vi "SystemController.UIClosed.vi"(8 "error in (no error)":errorcluster, 10 "UIClosed":T1, 11 "SystemController":refnum<class "SystemController.lvclass">) -> (0 "error out":errorcluster, 3 "SystemController out":refnum<class "SystemController.lvclass">)   [LabVIEW 2017, in "SystemController.lvclass"]
doc: "---------------------------------------------------------------\nJKI State Machine Objects™\nhttp://jki.net/state-machine-objects/\nCopyright (C) 2005-2015, JKI <info@jki.net>\nALL RIGHTS RESERVEDJKI State Machine Objects (SMO) 1.0.0.4\nJKI - JKI\nCopyright (c) 2015, JKI"
uses:
  SystemController.lvclass
  Typedefs/PublicEvents--SystemController.UIClosed.ctl
  SystemController.lvclass/SystemController.ctl
panel:
  # "For instructions on how to use the JKI State Machine Objects, examples and video tutorials, visit:\nhttp://jki.net/state-machine-objects/\n\nJKI State Machine Objects™\nhttp://jki.net/state-machine-objects/\nCopyright (C) 2005-2015, JKI <info@jki.net>\nALL RIGHTS RESERVED"
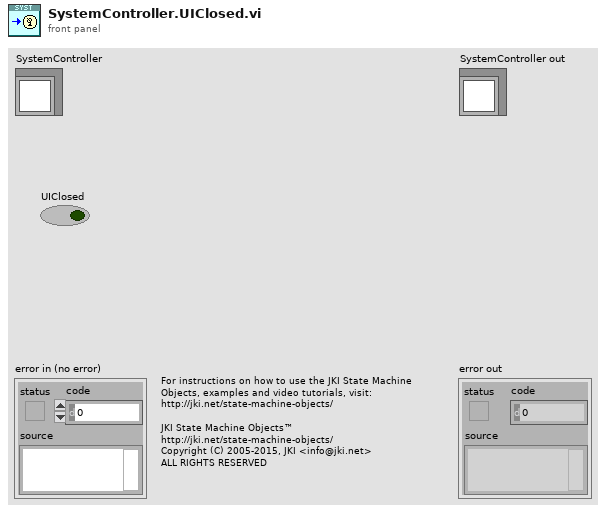
[diagram p1: front panel]
types:
  T1 = typedef "SystemController.lvclass/PublicEvents--SystemController.UIClosed.ctl" = bool
  T2 = typedef "SystemController.lvclass/PrivateData--Ref.ctl" = refnum<data-value>
  T3 = typedef "SystemController.lvclass/PrivateData--Cluster.ctl" = cluster{"Configuration":T4, "Dependencies":T8, "ProcessedImage":T9, "Public Events":T10}
  T4 = typedef "SystemController.lvclass/Configuration--Cluster.ctl" = cluster{"Camera":T5, "Find Eyes":bool, "Acquisition Rate (ms)":i32}
  T5 = typedef "SystemController.lvclass/CameraConfig--Cluster.ctl" = cluster{"Simulate Camera":bool, "IMAQ Camera":T6, "Simulated Camera Image":path}
  T6 = typedef "Camera_IMAQdx.lvclass/Configuration--Cluster.ctl" = cluster{"Camera Interface Name":string, "Number of Buffers":u32, "Image Name":string, "Image Type":T7}
  T7 = typedef "Image Type" = u32
  T8 = typedef "SystemController.lvclass/Dependencies--Cluster.ctl" = cluster{"Camera":refnum<class "Camera.lvclass">, "ImageFacialDetection":refnum<class "ImageFacialDetection.lvclass">}
  T9 = typedef "IMAQ Image.ctl" = refnum<image>
  T10 = typedef "SystemController.lvclass/PublicEvents--Cluster.ctl" = cluster{"UIClosed":refnum<user-event>}
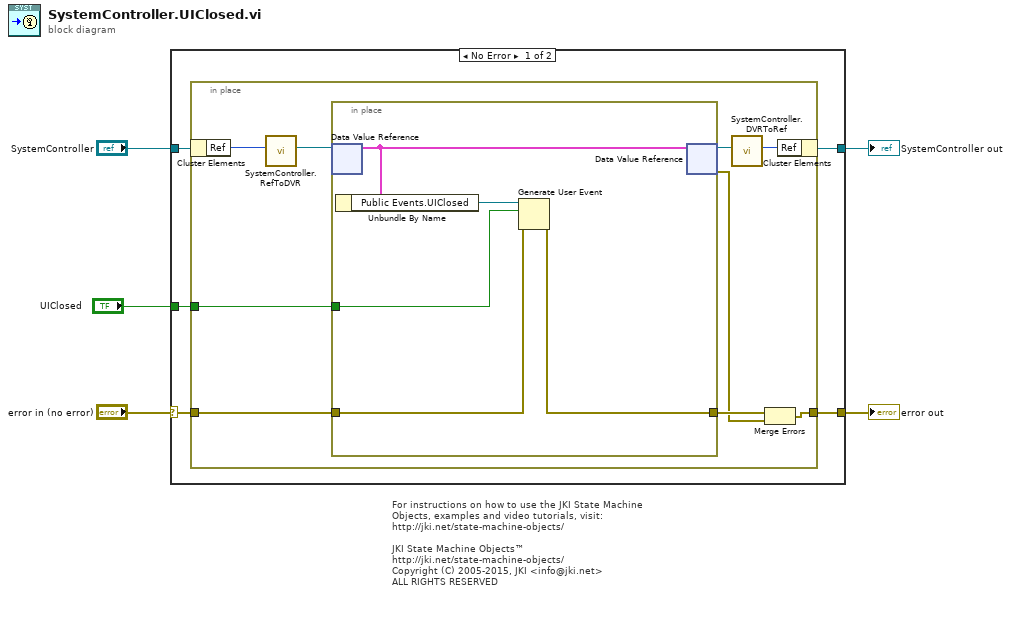
[diagram p0: block diagram]
diagram:
  # "For instructions on how to use the JKI State Machine Objects, examples and video tutorials, visit:\nhttp://jki.net/state-machine-objects/\n\nJKI State Machine Objects™\nhttp://jki.net/state-machine-objects/\nCopyright (C) 2005-2015, JKI <info@jki.net>\nALL RIGHTS RESERVED"
  n1 = case shown="No Error" "error in (no error)" {
    selector: "error in (no error)" -> [w8 w26]
    tunnel: [w7 w26] -> w4
    tunnel: [w9 w25] -> w5
    tunnel: "SystemController" -> [w10 w25]
    tunnel: "UIClosed" -> [w6 _]
    frame No Error {
      n2 = in-place {
        in-place-border: w8 -> [w19]
        in-place-border: [w16] -> w7
        in-place-border: w6 -> [w13]
        n3 = in-place-cluster #1(w10) -> ("Ref"=w15:u32)
        n4 = call "SystemController.RefToDVR.vi"("Ref"=w15) -> ("Ref"=w12:T2)  [unwired: 10 in]
        n5 = in-place {
          in-place-border: w19 -> [w22]
          in-place-border: [w21] -> w18
          in-place-border: w13 -> [w20]
          n6 = in-place-dvr #2(w12) -> (w24:T3)  [unwired: 1 out]
          n7 = Unbundle By Name(w24) -> ("Public Events.UIClosed"=w23:refnum<user-event>)
          n8 = Generate User Event(user event=w23, event data cluster=w20, error in=w22) -> (error out=w21:errorcluster)  [unwired: 1 in, 1 out]
          n9 = in-place-dvr #2(w24) -> (w14:T2, w17:errorcluster)
        }
        n10 = call "SystemController.DVRToRef.vi"("Ref"=w14) -> ("Ref"=w11:u32)  [unwired: 10 in]
        n11 = Merge Errors(w18, w17) -> (w16:errorcluster)
        n12 = in-place-cluster #1("Ref"=w11) -> (w9:refnum<class "SystemController.lvclass">)
      }
    }
    frame Error {
    }
  }
  "error out" <- w4
  "SystemController out" <- w5
